vi "Remove test suites.vi"(6 "Linker.Read Info From File":T2(array[cluster]), 9 "Define Test index":i32, 10 "Define Test Suite index":i32, 11 "Directory to search":path) -> (3 "Tests":path[](array[path]))   [LabVIEW 2013, in "Caraya.lvlib" / "Test Runner.lvclass"]
uses:
  Test Runner.lvclass
  <vilib>/Utility/lvfile.llb/LVFileType.ctl
  <vilib>/Utility/lvfile.llb/NI_FileType.lvlib
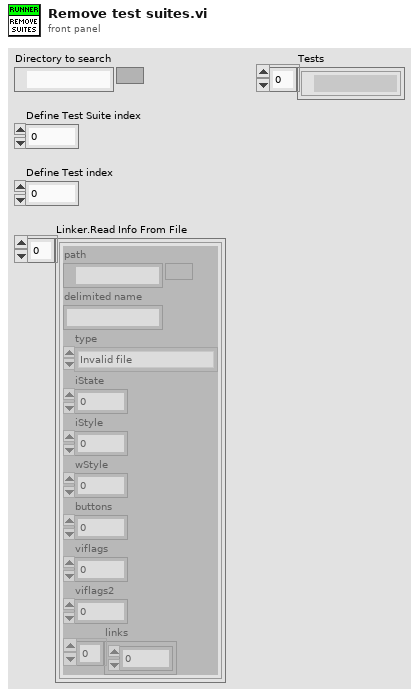
[diagram p1: front panel]
types:
  T1 = typedef "NI_FileType.lvlib/LVFileType.ctl" = enum32{"Invalid file", "Unknown type", "Instrument", "Control", "Polymorphic VI", "Project", "Library", "LVClass", "XControl", "XNode", "Shared library", ".NET assembly", "ActiveX interface", "CIN", "Run-time menu", "Palette menu", "Help file", "LLB", "XNode Edit Dependency", "Class Private Data Control", "Statechart", "MathScript .m file", "Ladder Diagram", "LVLibp", "XNode Build Dependency"}
  T2 = cluster{"path":path, "delimited name":string, "type":T1, "iState":u32, "iStyle":u16, "wStyle":u16, "buttons":u16, "viflags":u32, "viflags2":u32, "links":u32[]}[]
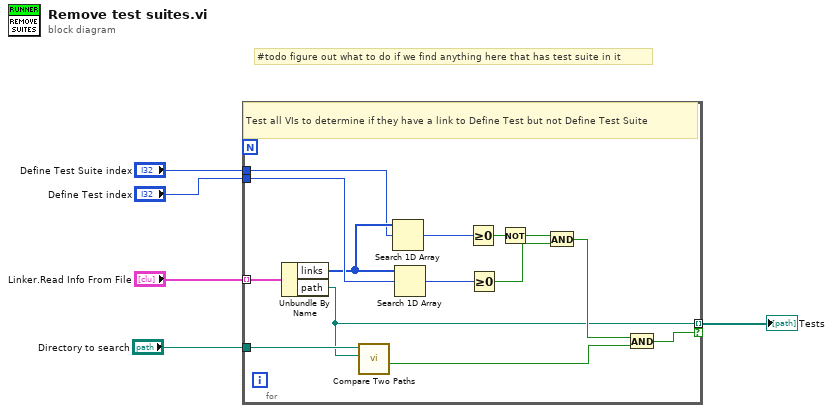
[diagram p0: block diagram]
diagram:
  # "#todo figure out what to do if we find anything here that has test suite in it"
  n1 = for {
    tunnel: "Linker.Read Info From File" -> [w19] mode=indexing
    tunnel: "Define Test Suite index" -> [w16]
    tunnel: "Define Test index" -> [w18]
    tunnel: [w8] -> w5 mode=indexing if=w7
    tunnel: "Directory to search" -> [w9]
    # "Test all VIs to determine if they have a link to Define Test but not Define Test Suite"
    n2 = Unbundle By Name(w19) -> ("links"=w17:u32[], "path"=w8:path)
    n3 = call <vilib>:"Compare Two Paths.vi"("Path 2"=w8, "Path 1"=w9) -> ("Path 2 Relative to Path 1?"=w6:bool)  [unwired: 6 in, 3 out]
    n4 = Search 1D Array(1D array=w17, element=w16) -> (index of element=w15:i32)  [unwired: 1 in]
    n5 = Search 1D Array(1D array=w17, element=w18) -> (index of element=w14:i32)  [unwired: 1 in]
    n6 = Greater Or Equal To 0?(x=w15) -> (x >= 0?=w11:bool)
    n7 = Greater Or Equal To 0?(x=w14) -> (x >= 0?=w12:bool)
    n8 = Not(x=w11) -> (.not. x?=w10:bool)
    n9 = And(x=w10, y=w12) -> (x .and. y?=w13:bool)
    n10 = And(x=w13, y=w6) -> (x .and. y?=w7:bool)
  }
  "Tests" <- w5
